vi "Write Configured.vi"(8 "error in":errorcluster, 10 "Configured?":bool, 11 "Instrument in":refnum<class "Instrument.lvclass">) -> (0 "error out":errorcluster, 3 "Instrument out":refnum<class "Instrument.lvclass">)   [LabVIEW 2012, in "Instrument.lvclass"]
doc: "Set the <b>Configured?</b> property. If there is an error in, this property will be set to FALSE and should be properly handled downstream."
uses:
  Instrument.lvclass
  Instrument.lvclass/Instrument.ctl
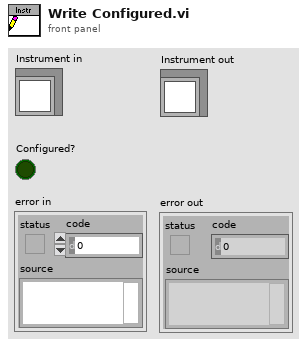
[diagram p1: front panel]
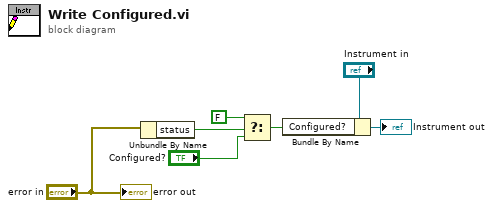
[diagram p0: block diagram]
diagram:
  n1 = Unbundle By Name("error in") -> ("status"=w5:bool)
  n2 = Select(t=FALSE, s=w5, f="Configured?") -> (s? t:f=w2:bool)
  n3 = Bundle By Name(cluster="Instrument in", "Configured?"=w2) -> (→"Instrument out":refnum<class "Instrument.lvclass">)
  "error out" <- "error in"
